vi "Reset.vi"(0 "VISA resource name":refnum<visa-resource-name>, 5 "error in (no error)":errorcluster) -> (14 "VISA resource name out":refnum<visa-resource-name>, 19 "error out":errorcluster)   [LabVIEW 2020, in "Keithley 2100 Series.lvlib"]
doc: "This VI resets the instrument, and then sends a set of default setup commands to the instrument."
uses:
  Keithley 2100 Series.lvlib
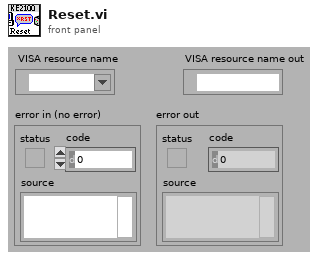
[diagram p1: front panel]
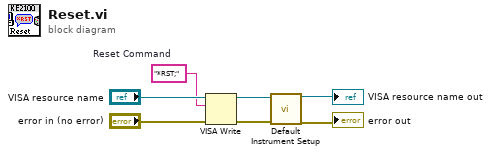
[diagram p0: block diagram]
diagram:
  w5 = "*RST;"  # Reset Command
  n1 = VISA Write(VISA resource name="VISA resource name", write buffer=w5, error in (no error)="error in (no error)") -> (VISA resource name out=w4:refnum<visa-resource-name>, error out=w3:errorcluster)  [unwired: 1 out]
  n2 = call "Default Instrument Setup.vi"("VISA resource name"=w4, "error in (no error)"=w3) -> ("VISA resource name out"=→"VISA resource name out":refnum<visa-resource-name>, "error out"=→"error out":errorcluster)  [unwired: 16 in]
